vi "AOL Z Cal-Emergency cal source.vi"() -> (0 "error out":errorcluster={"status"=TRUE, "code"=5001, "source"="Failed to load Motor Z Calibration"}, 1 "FOV Sizes":dbl[](array[numeric]), 2 "Calibration Data":dbl[][](array[numeric]))   [LabVIEW 2017]
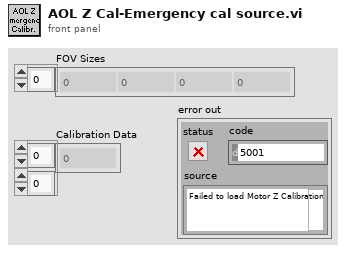
[diagram p1: front panel]
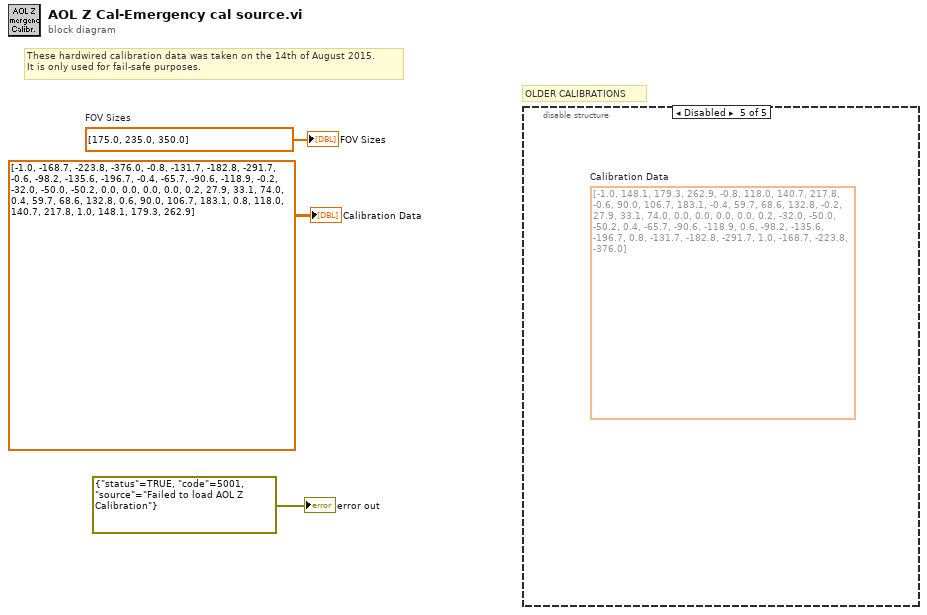
[diagram p0: block diagram]
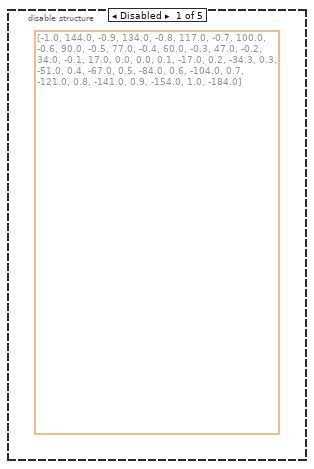
[diagram p2: hidden frame]
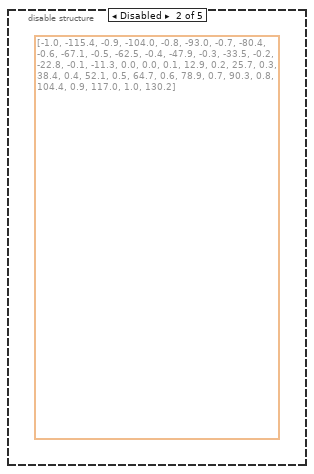
[diagram p3: hidden frame]
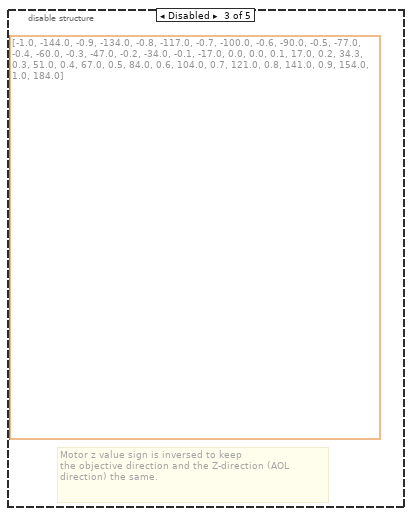
[diagram p4: hidden frame]
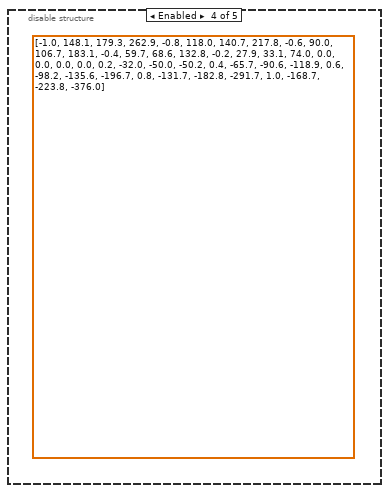
[diagram p5: hidden frame]
diagram:
  w3 = dbl[] [175.0, 235.0, 350.0]  # FOV Sizes
  # "OLDER CALIBRATIONS"
  # "These hardwired calibration data was taken on the 14th of August 2015.\nIt is only used for fail-safe purposes."
  n1 = disable-structure shown="Disabled" {
    frame Disabled {
      (unwired) dbl[][] [[-1.0, 144.0], [-0.9, 134.0], [-0.8, 117.0], [-0.7, 100.0], [-0.6, 90.0], [-0.5, 77.0], [-0.4, 60.0], [-0.3, 47.0], [-0.2, 34.0], [-0.1, 17.0], [0.0, 0.0], [0.1, -17.0], [0.2, -34.3], [0.3, -51.0], [0.4, -67.0], [0.5, -84.0], [0.6, -104.0], [0.7, -121.0], [0.8, -141.0], [0.9, -154.0], [1.0, -184.0]]
    }
    frame Disabled {
      (unwired) dbl[][] [[-1.0, -115.4], [-0.9, -104.0], [-0.8, -93.0], [-0.7, -80.4], [-0.6, -67.1], [-0.5, -62.5], [-0.4, -47.9], [-0.3, -33.5], [-0.2, -22.8], [-0.1, -11.3], [0.0, 0.0], [0.1, 12.9], [0.2, 25.7], [0.3, 38.4], [0.4, 52.1], [0.5, 64.7], [0.6, 78.9], [0.7, 90.3], [0.8, 104.4], [0.9, 117.0], [1.0, 130.2]]
    }
    frame Disabled {
      (unwired) dbl[][] [[-1.0, -144.0], [-0.9, -134.0], [-0.8, -117.0], [-0.7, -100.0], [-0.6, -90.0], [-0.5, -77.0], [-0.4, -60.0], [-0.3, -47.0], [-0.2, -34.0], [-0.1, -17.0], [0.0, 0.0], [0.1, 17.0], [0.2, 34.3], [0.3, 51.0], [0.4, 67.0], [0.5, 84.0], [0.6, 104.0], [0.7, 121.0], [0.8, 141.0], [0.9, 154.0], [1.0, 184.0]]
      # "Motor z value sign is inversed to keep\nthe objective direction and the Z-direction (AOL direction) the same."
    }
    frame Enabled {
      (unwired) dbl[][] [[-1.0, 148.1, 179.3, 262.9], [-0.8, 118.0, 140.7, 217.8], [-0.6, 90.0, 106.7, 183.1], [-0.4, 59.7, 68.6, 132.8], [-0.2, 27.9, 33.1, 74.0], [0.0, 0.0, 0.0, 0.0], [0.2, -32.0, -50.0, -50.2], [0.4, -65.7, -90.6, -118.9], [0.6, -98.2, -135.6, -196.7], [0.8, -131.7, -182.8, -291.7], [1.0, -168.7, -223.8, -376.0]] ("appended array")
    }
    frame Disabled {
      (unwired) dbl[][] [[-1.0, 148.1, 179.3, 262.9], [-0.8, 118.0, 140.7, 217.8], [-0.6, 90.0, 106.7, 183.1], [-0.4, 59.7, 68.6, 132.8], [-0.2, 27.9, 33.1, 74.0], [0.0, 0.0, 0.0, 0.0], [0.2, -32.0, -50.0, -50.2], [0.4, -65.7, -90.6, -118.9], [0.6, -98.2, -135.6, -196.7], [0.8, -131.7, -182.8, -291.7], [1.0, -168.7, -223.8, -376.0]]  # Calibration Data
    }
  }
  "FOV Sizes" <- w3
  "Calibration Data" <- dbl[][] [[-1.0, -168.7, -223.8, -376.0], [-0.8, -131.7, -182.8, -291.7], [-0.6, -98.2, -135.6, -196.7], [-0.4, -65.7, -90.6, -118.9], [-0.2, -32.0, -50.0, -50.2], [0.0, 0.0, 0.0, 0.0], [0.2, 27.9, 33.1, 74.0], [0.4, 59.7, 68.6, 132.8], [0.6, 90.0, 106.7, 183.1], [0.8, 118.0, 140.7, 217.8], [1.0, 148.1, 179.3, 262.9]] ("output array")
  "error out" <- errorcluster {"status"=TRUE, "code"=5001, "source"="Failed to load AOL Z Calibration"} ("error in (no error)")
